vi "Read Intake Current.vi"(8 "Proposed Power":dbl, 11 "Current":dbl) -> (1 "Actual Power":dbl, 2 "Forward Trip":bool, 3 "Backward Trip":bool)   [LabVIEW 2015]
uses:
  Common Code/Intake Current Trip States.ctl
  Robot Global Data.vi
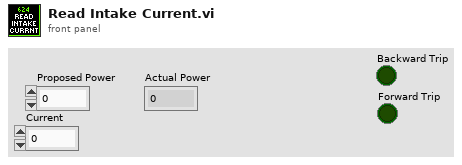
[diagram p1: front panel]
types:
  T1 = typedef "Intake Current Trip States.ctl" = enum16{"Normal", "Backward Trip", "Forward Trip"}
  T2 = typedef "Dashboard Control Data.ctl" = cluster{"Encoder Control":T3, "Steer PID output":cluster{"output high":dbl, "output low":dbl}, " Steer PID gains":cluster{"proportional gain (Kc)":dbl, "integral time (Ti, min)":dbl, "derivative time (Td, min)":dbl}, "Drivetrain Settings":T4, "Vision Packet":T5, "Dashboard Drivetrain Command":T6, "Info/Command Cluster":T8, "Ball Vision Packet":T9, "Intake Presets":T11, "Intake Encoder Control":T13, "Goal Output Range":cluster{"output high":dbl, "output low":dbl}, "Enabled Systems":T14, "Auton Presets":T15, "Pressure M":dbl, "Pressure B":dbl, "Vision Timeout":dbl, "Auto-Shift":T16, "Catapult Setpoints":T17, "Climb Presets":T18}
  T3 = typedef "Encoder Control.ctl" = cluster{"Right Tick Constant":dbl, "Left Tick Constant":dbl, "Reset?":bool, "Y Dist":cluster{"PID gains":cluster{"proportional gain (Kc)":dbl, "integral time (Ti, min)":dbl, "derivative time (Td, min)":dbl}}, "Y Stop Thresh":dbl, "Y Stop Speed":dbl}
  T4 = typedef "Drivetrain Settings.ctl" = cluster{"Gyro Tolerance":dbl, "Throttle Ramp (ms)":dbl, "Kv":dbl, "Ka":dbl, "Feed Forward P":dbl, "Feed Forward D":dbl, "Goal Vision PID gains":cluster{"proportional gain (Kc)":dbl, "integral time (Ti, min)":dbl, "derivative time (Td, min)":dbl}, "Goal Detection Window":dbl, "Creep Rate":dbl, "Vision Throttle Threshold":dbl, "Min Turn Output":dbl, "Left Batter Angle":dbl, "Right Batter Angle":dbl}
  T5 = typedef "Goal Vision Packet.ctl" = cluster{"Distance":dbl, "Center X":dbl, "Center Y":dbl, "Found Target?":bool, "Robot Center":dbl, "Angle":dbl}
  T6 = typedef "Dashboard Drivetrain Command.ctl" = cluster{"Drivetrain Vision":T7}
  T7 = typedef "Drivetrain Vision.ctl" = cluster{"Goal Window":dbl, "Ball Window":dbl}
  T8 = typedef "Ball Tracking Command Cluster.ctl" = cluster{"Distance to Ball":dbl, "Desired Angle":dbl, "Command":enum16{"Turn to Ball", "Turn to Angle", "Get Distance"}, "Pixels from Center":dbl}
  T9 = typedef "Ball Vision Packet.ctl" = cluster{"Ball Detected?":bool, "Distance to Ball":dbl, "Desired Angle":dbl, "Pixels from Center":dbl, "Tracking mode":T10}
  T10 = typedef "Tracking Mode.ctl" = enum16{"Turn to Ball", "Turn to Angle"}
  T11 = typedef "Intake Presets.ctl" = cluster{"Intake Speed":dbl, "Outake Speed":dbl, "Angle Speed":dbl, "Angle Tolerance":dbl, "Encoder Scale":dbl, "Load Height":dbl, "Output Range":T12, "MaxCurrent":dbl, "Idle Height":dbl, "Max Height":dbl, "Reset Encoders?":bool, "PID gains":cluster{"proportional gain (Kc)":dbl, "integral time (Ti, min)":dbl, "derivative time (Td, min)":dbl}, "Drop Low Height ":dbl, "Rotation Power Max/Min":dbl, "Reset Delay":dbl}
  T12 = typedef "Drivetrain Output Range.ctl" = cluster{"output high":dbl, "output low":dbl}
  T13 = typedef "IntakeEcoderControl.ctl" = cluster{"Arm Tick Constant":dbl, "Reset?":bool, "Y Dist":cluster{"PID gains":cluster{"proportional gain (Kc)":dbl, "integral time (Ti, min)":dbl, "derivative time (Td, min)":dbl}}, "Y Stop Thresh":dbl, "Y Stop Speed":dbl}
  T14 = typedef "Enabled Systems.ctl" = cluster{"Shoot":bool, "Intake":bool, "DT":bool, "Gyro":bool, "100ms":bool, "US":bool}
  T15 = typedef "Autonomous Presets.ctl" = cluster{"Pitch Limit":dbl, "Roll Limit":dbl, "Start Position":dbl, "Cross Position":dbl}
  T16 = typedef "Auto Shift Cluster.ctl" = cluster{"Delay":dbl, "Speed Thresh":dbl, "Upshift Accel":dbl, "Upshift Throttle":dbl, "Upshift Throttle Accel":dbl, "Downshift Throttle":dbl, "Downshift Throttle Accel":dbl, "Pressure Threshold":dbl}
  T17 = typedef "Catapult Presets.ctl" = cluster{"Intake Danger Height":dbl, "Ball Security Delay ":dbl, "High PSI Minimum":dbl, "Shot Finish Delay":dbl, "Low PSI Minimum":dbl, "Idle Ball Security Wait ":dbl}
  T18 = typedef "Climb Presets.ctl" = cluster{"Winch Speed":dbl}
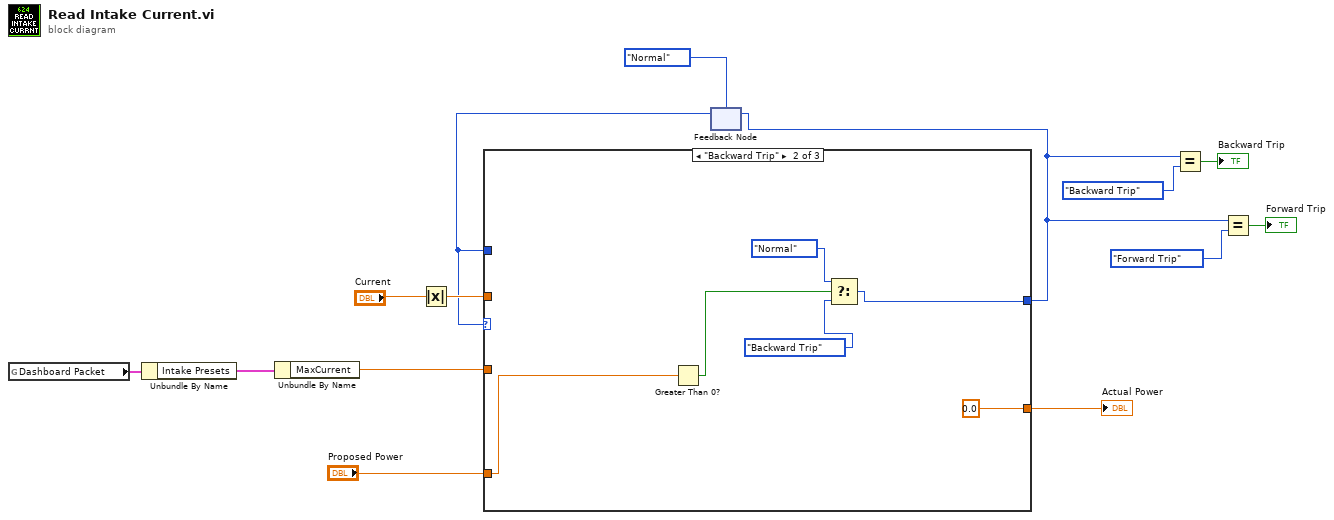
[diagram p0: block diagram]
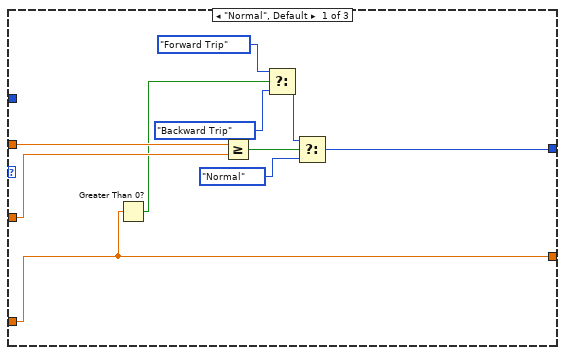
[diagram p2: hidden frame]
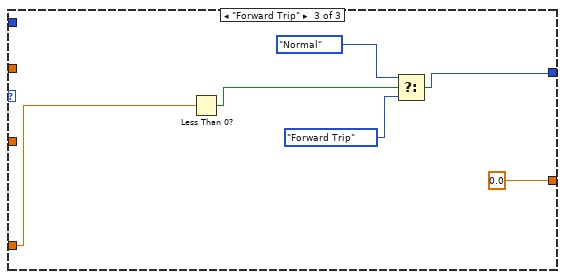
[diagram p3: hidden frame]
diagram:
  n1 = global read "Robot Global Data.vi" "Dashboard Packet"() -> (w14:T2)
  n2 = Unbundle By Name(w14) -> ("Intake Presets"=w13:T11)
  n3 = Unbundle By Name(w13) -> ("MaxCurrent"=w11:dbl)
  n4 = Absolute Value(x="Current") -> (abs(x)=w10:dbl)
  n5 = feedback #1(Intake_Current_Trip_States."Normal" ("Current Trip States")) -> (w1:T1)
  n6 = case shown="\"Backward Trip\"" w1 {
    tunnel: w1 -> [_ _ _]
    tunnel: "Proposed Power" -> [w16 w27 w33]
    tunnel: [w16 0.0 0.0] -> w2
    tunnel: w11 -> [w23 _ _]
    tunnel: w10 -> [w24 _ _]
    tunnel: [w17 w28 w34] -> w5
    frame "Normal", Default {
      n7 = Greater Than 0?(x=w16) -> (x > 0?=w15:bool)
      n8 = Greater Or Equal?(x=w24, y=w23) -> (x >= y?=w22:bool)
      n9 = Select(t=Intake_Current_Trip_States."Forward Trip" ("Current Trip States"), s=w15, f=Intake_Current_Trip_States."Backward Trip" ("Current Trip States")) -> (s? t:f=w21:T1)
      n10 = Select(t=w21, s=w22, f=Intake_Current_Trip_States."Normal" ("Current Trip States")) -> (s? t:f=w17:T1)
    }
    frame "Backward Trip" {
      n11 = Greater Than 0?(x=w27) -> (x > 0?=w26:bool)
      n12 = Select(t=Intake_Current_Trip_States."Normal" ("Current Trip States"), s=w26, f=Intake_Current_Trip_States."Backward Trip" ("Current Trip States")) -> (s? t:f=w28:T1)
    }
    frame "Forward Trip" {
      n13 = Less Than 0?(x=w33) -> (x < 0?=w32:bool)
      n14 = Select(t=Intake_Current_Trip_States."Normal" ("Current Trip States"), s=w32, f=Intake_Current_Trip_States."Forward Trip" ("Current Trip States")) -> (s? t:f=w34:T1)
    }
  }
  "Actual Power" <- w2
  n15 = feedback-in #1(w5) -> ()
  n16 = Equal?(x=w5, y=Intake_Current_Trip_States."Backward Trip" ("Current Trip States")) -> (x = y?=→"Backward Trip":bool)
  n17 = Equal?(x=w5, y=Intake_Current_Trip_States."Forward Trip" ("Current Trip States")) -> (x = y?=→"Forward Trip":bool)
